vi "Harmonics MSMT Set DC Params.vi"(8 "error in (no error)":errorcluster, 10 "Step In":refnum<k7>, 11 "Harmonics in":refnum<class "Harmonics.lvclass">) -> (0 "error out":errorcluster, 2 "Step Out":refnum<k7>, 3 "Harmonics out":refnum<class "Harmonics.lvclass">)   [LabVIEW 2018, in "Harmonics.lvlib" / "Harmonics.lvclass"]
uses:
  Harmonics.lvclass
  Harmonics.lvclass/Harmonics.ctl
  Read DC Pins.vi
  Plugins/TestStand API Tools (TSAT).lvlibp/Step Actions/TSAT Step Actions.lvlib
  C:/Sequence Automation/Plugins/Measurement Interface.lvlibp/Measurement Interface.lvclass
  Plugins/Measurement Interface.lvlibp/Measurement Interface.lvclass
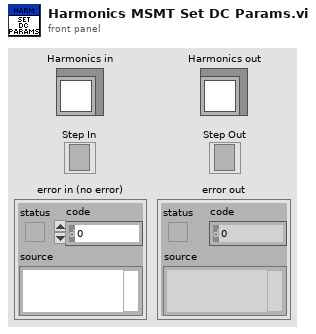
[diagram p1: front panel]
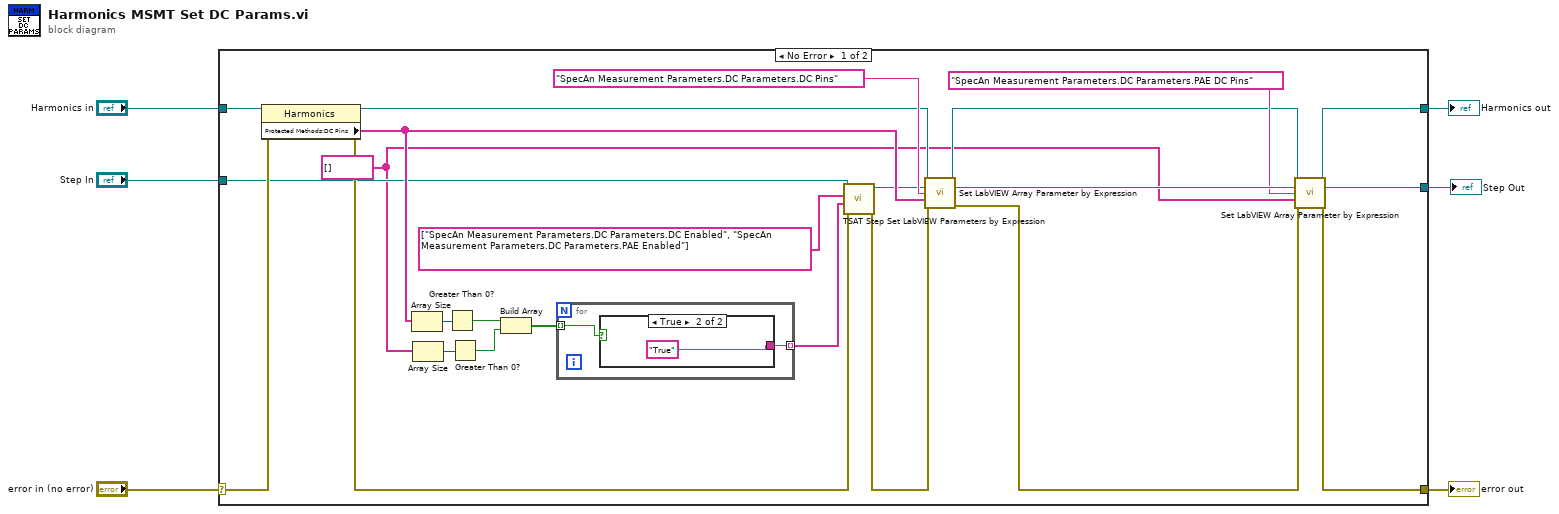
[diagram p0: block diagram]
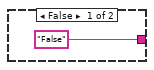
[diagram p2: hidden frame]
diagram:
  n1 = case shown="No Error" "error in (no error)" {
    selector: "error in (no error)" -> [w11 w37]
    tunnel: [w10 w37] -> w5
    tunnel: [w12 w36] -> w3
    tunnel: "Harmonics in" -> [w13 w36]
    tunnel: "Step In" -> [w9 w35]
    tunnel: [w8 w35] -> w1
    frame No Error {
      w7 = string[] [] ("Array of Expresssions")
      n2 = property class="Harmonics"(reference=w13, error in=w11) -> (reference out=w26:refnum<class "Harmonics.lvclass">, error out=w23:errorcluster, "Protected Methods:DC Pins"=w24:string[])
      n3 = Array Size(array=w24) -> (size(s)=w21:i32)
      n4 = Array Size(array=w7) -> (size(s)=w20:i32)
      n5 = Greater Than 0?(x=w21) -> (x > 0?=w19:bool)
      n6 = Greater Than 0?(x=w20) -> (x > 0?=w18:bool)
      n7 = Build Array(w19, w18) -> (w17:bool[])
      n8 = for {
        tunnel: w17 -> [w32] mode=indexing
        tunnel: [w31] -> w16 mode=indexing
        n9 = case shown="True" w32 {
          tunnel: ["False" "True"] -> w31
          frame False {
          }
          frame True {
          }
        }
      }
      n10 = call "TSAT Step Set LabVIEW Parameters by Expression.vi"("Error In"=w23, "Value Expressions"=w16, "Parameters to Set"=string[] ["SpecAn Measurement Parameters.DC Parameters.DC Enabled", "SpecAn Measurement Parameters.DC Parameters.PAE Enabled"], "Step In"=w9) -> ("Error Out"=w22:errorcluster, "Step Out"=w15:refnum<k7>)  [unwired: 6 in]
      n11 = call "Set LabVIEW Array Parameter by Expression.vi"("Measurement Interface in"=w26, "Step In"=w15, "LabVIEW Parameter to Set"="SpecAn Measurement Parameters.DC Parameters.DC Pins", "Array of Expresssions"=w24, "error in (no error)"=w22) -> ("Measurement Interface out"=w25:refnum<class "Harmonics.lvclass">, "Step Out"=w28:refnum<k7>, "error out"=w29:errorcluster)  [unwired: 8 in]
      n12 = call "Set LabVIEW Array Parameter by Expression.vi"("Measurement Interface in"=w25, "Step In"=w28, "LabVIEW Parameter to Set"="SpecAn Measurement Parameters.DC Parameters.PAE DC Pins", "Array of Expresssions"=w7, "error in (no error)"=w29) -> ("Measurement Interface out"=w12:refnum<class "Harmonics.lvclass">, "Step Out"=w8:refnum<k7>, "error out"=w10:errorcluster)  [unwired: 8 in]
    }
    frame Error {
    }
  }
  "error out" <- w5
  "Harmonics out" <- w3
  "Step Out" <- w1
